vi "Untitled 2.vi"() -> ()   [LabVIEW 2014]
panel:
  in  "Y":dbl[](array[numeric])
  in  "X":dbl[](array[numeric])
  in  "T3 positioning test range (V)":T1
  out "Intensity Graph":dbl[][](graph)
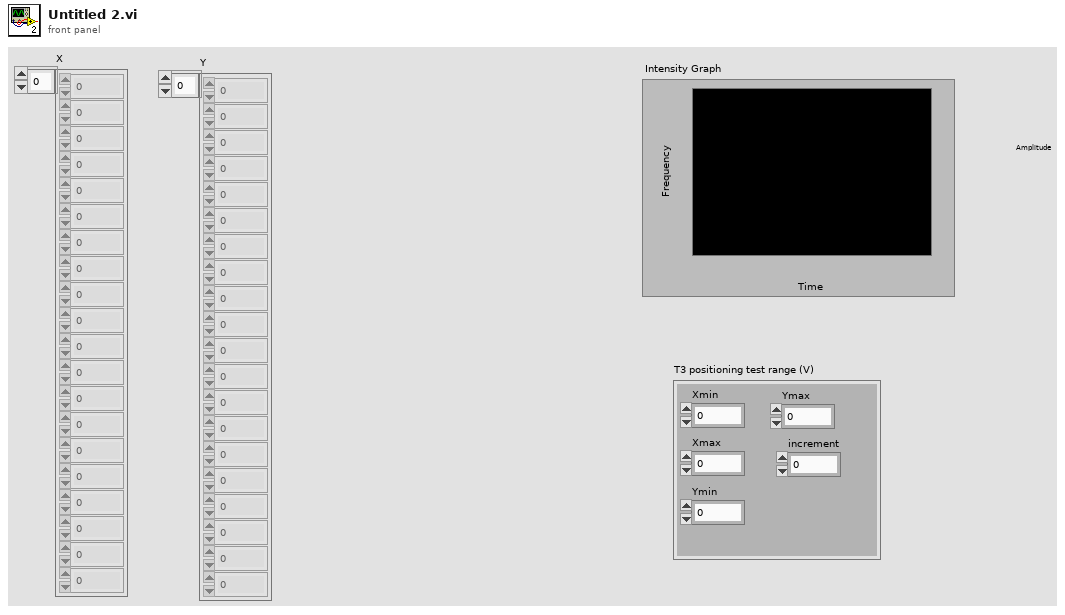
[diagram p1: front panel]
types:
  T1 = cluster{"Xmin":dbl, "Xmax":dbl, "Ymin":dbl, "Ymax":dbl, "increment":dbl}
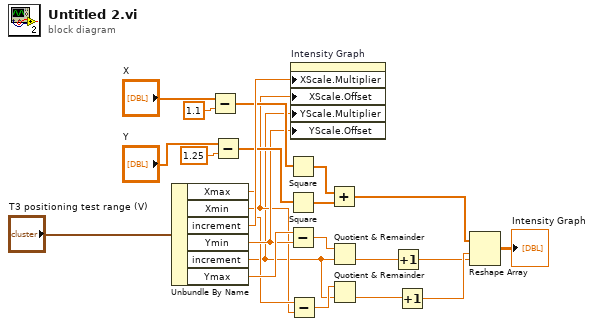
[diagram p0: block diagram]
diagram:
  n1 = Unbundle By Name("T3 positioning test range (V)") -> ("Xmax"=w8:dbl, "Xmin"=w7:dbl, "increment"=w22:dbl, "Ymin"=w12:dbl, "increment"=w5:dbl, "Ymax"=w13:dbl)
  n2 = Subtract(x="X", y=1.1) -> (x-y=w16:dbl[])
  n3 = Subtract(x="Y", y=1.25) -> (x-y=w17:dbl[])
  n4 = Square(x=w16) -> (x^2=w15:dbl[])
  n5 = Square(x=w17) -> (x^2=w14:dbl[])
  n6 = Subtract(x=w13, y=w12) -> (x-y=w11:dbl)
  n7 = Subtract(x=w8, y=w7) -> (x-y=w6:dbl)
  n8 = property on="Intensity Graph" class="IntGraph (strict)"("XScale.Multiplier"=w22, "XScale.Offset"=w7, "YScale.Multiplier"=w5, "YScale.Offset"=w12) -> ()  [unwired: 2 in, 2 out]
  n9 = Add(x=w15, y=w14) -> (x+y=w10:dbl[])
  n10 = Quotient & Remainder(x=w11, y=w5) -> (floor(x/y)=w2:dbl)  [unwired: 1 out]
  n11 = Quotient & Remainder(x=w6, y=w5) -> (floor(x/y)=w4:dbl)  [unwired: 1 out]
  n12 = Increment(x=w2) -> (x+1=w1:dbl)
  n13 = Increment(x=w4) -> (x+1=w3:dbl)
  n14 = Reshape Array(w10, w3, w1) -> (→"Intensity Graph":dbl[][])
